vi "Find Project Target.vi"(8 "error in (no error)":errorcluster, 10 "Target Name":string, 11 "Project Sync Tools in":refnum<class "Project Sync Tools.lvclass">) -> (0 "error out":errorcluster, 1 "Found ?":bool, 2 "TargetItem out":refnum<vi>, 3 "Project Sync Tools out":refnum<class "Project Sync Tools.lvclass">)   [LabVIEW 2019, in "Project Sync Tools.lvclass"]
uses:
  Project Sync Tools.lvclass
  Project Sync Tools.lvclass/Project Sync Tools.ctl
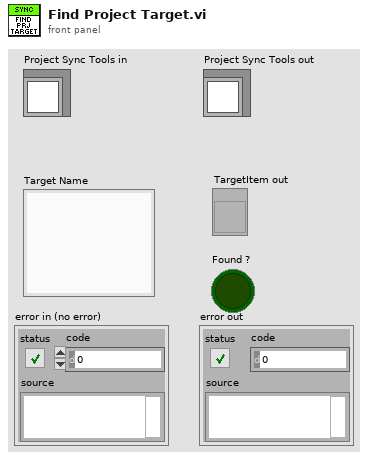
[diagram p1: front panel]
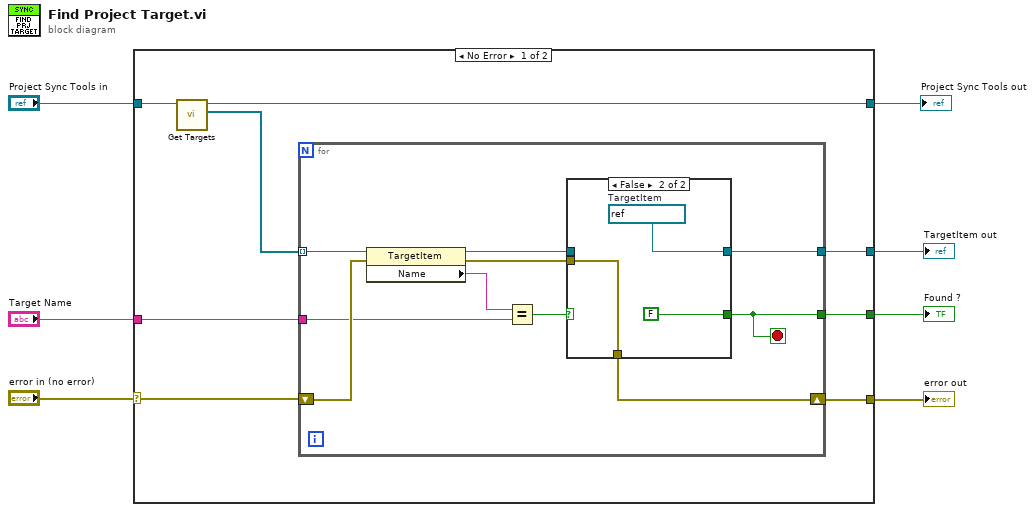
[diagram p0: block diagram]
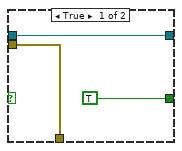
[diagram p2: hidden frame]
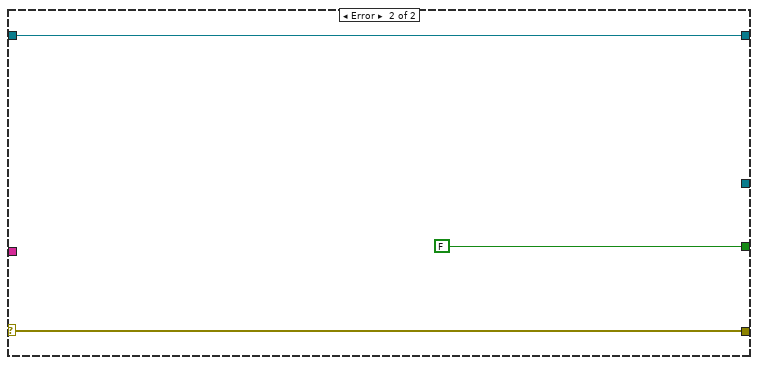
[diagram p3: hidden frame]
diagram:
  n1 = case shown="No Error" "error in (no error)" {
    selector: "error in (no error)" -> [w8 w33]
    tunnel: "Target Name" -> [w15 _]
    tunnel: [w14 w33] -> w6
    tunnel: [w13 FALSE] -> w5
    tunnel: [w12 _] -> w3
    tunnel: "Project Sync Tools in" -> [w11 w32]
    tunnel: [w10 w32] -> w1
    frame No Error {
      n2 = call "Get Targets.vi"("Project Sync Tools in"=w11) -> ("Targets"=w9:refnum<vi>[], "Project Sync Tools out"=w10:refnum<class "Project Sync Tools.lvclass">)  [unwired: 9 in]
      n3 = for {
        shift-right: [w23] -> w14
        shift-left: w8 -> [w25]
        tunnel: w15 -> [w20]
        tunnel: [w21] -> w13
        tunnel: [w22] -> w12
        tunnel: w9 -> [w17] mode=indexing
        stop <- w21 stop-if-true
        n4 = property class="TargetItem"(reference=w17, error in=w25) -> (reference out=w16:refnum<vi>, error out=w24:errorcluster, "Name"=w18:string)
        n5 = Equal?(x=w18, y=w20) -> (x = y?=w19:bool)
        n6 = case shown="False" w19 {
          tunnel: w24 -> [w28 w30]
          tunnel: [w28 w30] -> w23
          tunnel: [w26 w29] -> w22
          tunnel: [TRUE FALSE] -> w21
          tunnel: w16 -> [w26 _]
          frame True {
          }
          frame False {
            w29 = refnum<vi> refnum  # TargetItem
          }
        }
      }
    }
    frame Error {
    }
  }
  "TargetItem out" <- w3
  "error out" <- w6
  "Found ?" <- w5
  "Project Sync Tools out" <- w1
